vi "ProdaNG.WabcoNumber.Update.vi"(7 "newnWabcoNumber":string, 8 "error in":errorcluster, 9 "serialNumber":string, 10 "wabcoNumber":string, 11 "dbHandleIn":i32) -> (0 "error out":errorcluster, 3 "dbHandle":i32)   [LabVIEW 2016]
doc: "This function serves for identifying a system, if for example, the name and the Wabco Number of the tested part, or the process id and the sequential number in a process are known. \nParameter:\nhandle is an Integer, which is returned by the function Login() at the creation of a new connection.\nsystemName is the name of the system, as it is deposited in the database. If unknown, NULL must be passed.\nwabcoNumber is a known Wabco number in the database. If unknown, NULL must be passed.\nprocessSequence is the sequential Number in the process. If unknown, 0 must be passed.\nprocessId is the according process id. If unknown, 0 must be passed.\n\nmyIdent is a pointer on an identification structure, if the returncode is 0. The structure must be defined in the calling program. The function tries to identify the system definitely under the aid of the passed parameter, in order to return the resulting id's in MyIdent.\n\nThe function tries to identify the system from the following combinations of the parameter:\nsystemName, \nprocessId, \nsystemName and wabcoNumber, \nprocessId and processSequence \nor from all 4 parameter.\nThe more parameters are set, the bigger is the chance, that the system can be identified.\nReturncodes:\n0 No error\n< 0 ORACLE Error Code\n6 (ERROR_INVALID_HANDLE) in case of an invalid handle\n232 (ERROR_NO_DATA) in case that the system cannot be identified definitely."
uses:
  prodllNG.dll
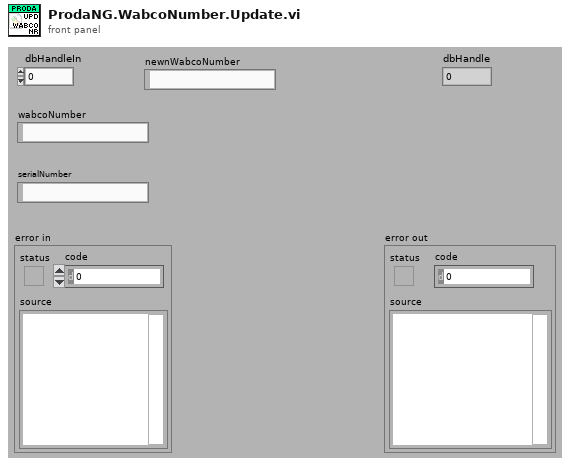
[diagram p1: front panel]
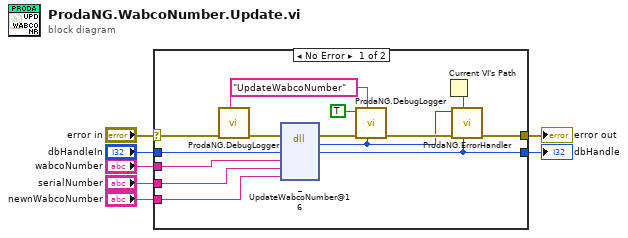
[diagram p0: block diagram]
diagram:
  n1 = case shown="No Error" "error in" {
    selector: "error in" -> [w17 w23]
    tunnel: [w21 w23] -> w6
    tunnel: [w12 w22] -> w5
    tunnel: "dbHandleIn" -> [w11 w22]
    tunnel: "wabcoNumber" -> [w10 _]
    tunnel: "serialNumber" -> [w9 _]
    tunnel: "newnWabcoNumber" -> [w8 _]
    frame No Error {
      w19 = "UpdateWabcoNumber" ("cmd")
      n2 = call "ProdaNG.DebugLogger.vi"("cmd"=w19, "error in (no error)"=w17) -> ("error out"=w16:errorcluster)  [unwired: 9 in]
      n3 = dll-call lib="D:/Maszup/WABCO/SVN/BSV/SOFTWARE-LASER/sources/Database/ProdaNG/prodllNG.dll" fn="_UpdateWabcoNumber@16" ("ProDll.dll:Login")(error in=w16, "dbHandle"=w11, "wabcoNumber"=w10, "serialNumber"=w9, "newWabcoNumber"=w8) -> (error out=w15:errorcluster, "return type"=w13:i32, "dbHandle"=w12:i32)  [unwired: 5 in, 1 out]
      n4 = call "ProdaNG.DebugLogger.vi"("return type"=w13, "cmd"=w19, "error in (no error)"=w15, "done? (F)"=TRUE) -> ("error out"=w14:errorcluster)  [unwired: 7 in]
      n5 = Current VI's Path() -> (path=w20:path)
      n6 = call "ProdaNG.ErrorHandler.vi"("dbHandleIn"=w12, "Path"=w20, "error in"=w14, "output_parameter"=w13) -> ("error out"=w21:errorcluster)  [unwired: 7 in]
    }
    frame Error {
    }
  }
  "error out" <- w6
  "dbHandle" <- w5
